vi "Standardize Multiple Angles in Degrees.vi"(3 "angles in (deg)":dbl[](array[numeric]), 4 "range (-180 to 180)":T1=enum."-180 to 180") -> (5 "angles out (deg)":dbl[](array[numeric]))   [LabVIEW 2017, in "NI_Robotics Utilities.lvlib"]
doc: "Wraps a 1D array of angles in degrees to be within a specific range.\n\nThis VI is deprecated. Use <vi.lib>\\Analysis\\coordinate.llb\\Wrap Angle.vi instead."
uses:
  <vilib>/robotics/Utilities/NI_Robotics Utilities.lvlib
  <vilib>/robotics/Utilities/Angle Range_Degrees.ctl
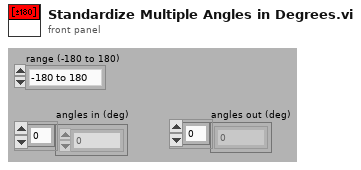
[diagram p1: front panel]
types:
  T1 = typedef "NI_Robotics Utilities.lvlib/Angle Range_Degrees.ctl" = enum16{"none", "-180 to 180", "0 to 360"}
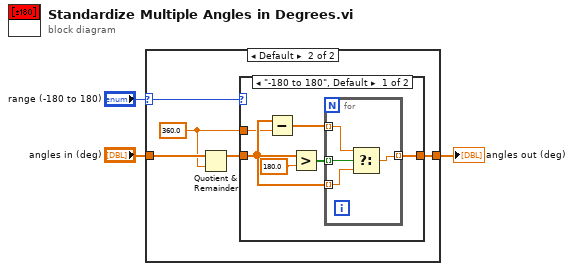
[diagram p0: block diagram]
diagram:
  n1 = case shown="Default" "range (-180 to 180)" {
    selector: "range (-180 to 180)" -> [_ w5]
    tunnel: "angles in (deg)" -> [w4 w9]
    tunnel: [w4 w8] -> w2
    frame "none" {
    }
    frame Default {
      w6 = 360.0
      n2 = Quotient & Remainder(x=w9, y=w6) -> (x-y*floor(x/y)=w7:dbl[])  [unwired: 1 out]
      n3 = case shown="\"-180 to 180\", Default" w5 {
        tunnel: [w15 w20] -> w8
        tunnel: w7 -> [w13 w20]
        tunnel: w6 -> [w11 _]
        frame "-180 to 180", Default {
          n4 = Subtract(x=w13, y=w11) -> (x-y=w12:dbl[])
          n5 = Greater?(x=w13, y=180.0) -> (0:w14:bool[])
          n6 = for {
            tunnel: w13 -> [w17] mode=indexing
            tunnel: w12 -> [w18] mode=indexing
            tunnel: [w16] -> w15 mode=indexing
            tunnel: w14 -> [w19] mode=indexing
            n7 = Select(t=w18, s=w19, f=w17) -> (s? t:f=w16:dbl)
          }
        }
        frame "0 to 360" {
        }
      }
    }
  }
  "angles out (deg)" <- w2
